vi "Write.vi"   [LabVIEW 2011, in "LVH-Adept.lvlib"]
doc: "Write data to a Digilent FPGA board that has been configured for use with the Adept interface."
uses:
  <vilib>/LabVIEW Hacker/Adept/LVH-Adept.lvlib
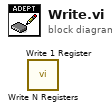
[diagram p0: block diagram]
diagram:
  n1 = call "Write N Registers.vi"() -> ()  [unwired: 10 in, 2 out]
  n2 = call "Write 1 Register.vi"() -> ()  [unwired: 10 in, 2 out]
